vi "rsscope_core_global.vi"() -> ()   [LabVIEW 2018] (continued)
all actions waiting for a trigger event. In particular, *TRG generates a manual trigger signal (Manual Trigger).\n\nAvailable Repeated Capabilities:\nNone\n\nRemote-control command(s):\n*TRG"}, {"Level"=2, "Class Only"=FALSE, "Identifier"="RSSCOPE_ATTR_SEND_SW_TRIGGER_AND_WAIT", "Descriptive Name"="Send SW Trigger And Wait", "Data Type"=4, "Command"="*TRG", "Access"=1, "Range Table"="", "Read Callback"="", "Write Callback"="", "Supported Models"="", "Instrument Options"="", "Flags"=1, "Help"="Triggers all actions waiting for a trigger event. In particular, *TRG generates a manual trigger signal (Manual Trigger). This attribute waits for operation complete.\n\nAvailable Repeated Capabilities:\nNone\n\nRemote-control command(s):\n*TRG"}, {"Level"=1, "Class Only"=TRUE, "Identifier"="", "Descriptive Name"="Cursors", "Data Type"=0, "Command"="", "Access"=0, "Range Table"="", "Read Callback"="", "Write Callback"="", "Supported Models"="", "Instrument Options"="", "Flags"=0, "Help"="Cursor measurements determine the results at the current cursor positions. The cursors can be positioned manually or can be configured to follow the peaks of the waveform. Up to four sets of cursors can be configured and displayed. Each set of cursors consists of a pair of horizontal or vertical cursors, or both. Cursors can be coupled so that the initially defined distance is always maintained."}, {"Level"=2, "Class Only"=FALSE, "Identifier"="RSSCOPE_ATTR_CURSOR_ENABLED", "Descriptive Name"="Cursor Enabled", "Data Type"=3, "Command"="CURS{Cursor}:STAT", "Access"=2, "Range Table"="", "Read Callback"="", "Write Callback"="", "Supported Models"="", "Instrument Options"="", "Flags"=0, "Help"="Switches the indicated cursor on or off.\n\nAvailable Repeated Capabilities:\nCursor: C1, C2, C3, C4\r\n\nRemote-control command(s):\nCURSor<m>:STATe"}, {"Level"=2, "Class Only"=FALSE, "Identifier"="RSSCOPE_ATTR_ALL_CURSORS_OFF", "Descriptive Name"="All Cursors Off", "Data Type"=4, "Command"="CURS1:AOFF", "Access"=1, "Range Table"="", "Read Callback"="", "Write Callback"="", "Supported Models"="", "Instrument Options"="", "Flags"=0, "Help"="Switches all cursors off.\n\nAvailable Repeated Capabilities:\nNone\n\nRemote-control command(s):\nCURSor<m>:AOFF"}, {"Level"=2, "Class Only"=FALSE, "Identifier"="RSSCOPE_ATTR_CURSOR_MEASUREMENT_TYPE", "Descriptive Name"="Cursor Measurement Type", "Data Type"=0, "Command"="CURS{Cursor}:FUNC", "Access"=2, "Range Table"="rsscope_rngCursorFunction", "Read Callback"="", "Write Callback"="", "Supported Models"="", "Instrument Options"="", "Flags"=0, "Help"="Defines the cursor measurement type.\n\nAvailable Repeated Capabilities:\nCursor: C1, C2, C3, C4\r\n\nRemote-control command(s):\nCURSor<m>:FUNCtion"}, {"Level"=2, "Class Only"=FALSE, "Identifier"="RSSCOPE_ATTR_CURSOR_SOURCE", "Descriptive Name"="Cursor Source", "Data Type"=0, "Command"="CURS{Cursor}:SOUR", "Access"=2, "Range Table"="RsScope_rngCursorSource", "Read Callback"="", "Write Callback"="", "Supported Models"="", "Instrument Options"="", "Flags"=0, "Help"="Defines the source of the cursor measurement.\n\nAvailable Repeated Capabilities:\nCursor: C1, C2, C3, C4\r\n\nRemote-control command(s):\nCURSor<m>:SOURce"}, {"Level"=2, "Class Only"=FALSE, "Identifier"="RSSCOPE_ATTR_CURSOR_TRACKING", "Descriptive Name"="Cursor Tracking", "Data Type"=3, "Command"="CURS{Cursor}:TRAC", "Access"=2, "Range Table"="", "Read Callback"="", "Write Callback"="", "Supported Models"="", "Instrument Options"="", "Flags"=0, "Help"="If set to ON, the horizontal cursor lines follow the waveform.\n\nAvailable Repeated Capabilities:\nCursor: C1, C2, C3, C4\r\n\nRemote-control command(s):\nCURSor<m>:TRACking[:STATe]"}, {"Level"=2, "Class Only"=FALSE, "Identifier"="RSSCOPE_ATTR_CURSOR_RESULT_TABLE_POSITION", "Descriptive Name"="Cursor Result Table Position", "Data Type"=0, "Command"="DISP:RES:CUP", "Access"=2, "Range Table"="RsScope_rngDisplayResultTableDefaultPosition", "Read Callback"="", "Write Callback"="", "Supported Models"="", "Instrument Options"="", "Flags"=0, "Help"="Defines the position of the cursor measurement results on the screen.\n\nAvailable Repeated Capabilities:\nNone\n\nRemote-control command(s):\nDISPlay:RESultboxes:CUPosition"}, {"Level"=2, "Class Only"=FALSE, "Identifier"="RSSCOPE_ATTR_CURSOR_X_POSITION_COUPLING", "Descriptive Name"="Cursor X Position Coupling", "Data Type"=3, "Command"="CURS{Cursor}:XCO", "Access"=2, "Range Table"="", "Read Callback"="", "Write Callback"="", "Supported Models"="", "Instrument Options"="", "Flags"=0, "Help"="Defines the positioning mode of the vertical cursor. \nON: Moving one cursor line moves the other cursor line too. The cursor lines always remain a fixed distance.\nOFF: Each cursor line is positioned independently.\n\nAvailable Repeated Capabilities:\nCursor: C1, C2, C3, C4\r\n\nRemote-control command(s):\nCURSor<m>:XCOupling"}, {"Level"=2, "Class Only"=FALSE, "Identifier"="RSSCOPE_ATTR_CURSOR_Y_POSITION_COUPLING", "Descriptive Name"="Cursor Y Position Coupling", "Data Type"=3, "Command"="CURS{Cursor}:YCO", "Access"=2, "Range Table"="", "Read Callback"="", "Write Callback"="", "Supported Models"="", "Instrument Options"="", "Flags"=0, "Help"="Defines the positioning mode of the horizontal cursor. If the horizontal cursor lines track the waveform, the y-coupling is irrelevant.\nON: Moving one cursor line moves the other cursor line too. The cursor lines always remain a fixed distance.\nOFF: Each cursor line is positioned independently.\n\nAvailable Repeated Capabilities:\nCursor: C1, C2, C3, C4\r\n\nRemote-control command(s):\nCURSor<m>:YCOupling"}, {"Level"=2, "Class Only"=FALSE, "Identifier"="RSSCOPE_ATTR_CURSOR_ENVELOPE_CURVE_1", "Descriptive Name"="Cursor Envelope Curve 1", "Data Type"=0, "Command"="CURS{Cursor}:X1EN", "Access"=2, "Range Table"="rsscope_rngMinMax", "Read Callback"="", "Write Callback"="", "Supported Models"="", "Instrument Options"="", "Flags"=0, "Help"="If the waveform arithmetics are set to envelope curve and cursor tracking is set to &apos;ON&apos;, this setting defines how the first horizontal cursor is positioned.\n\nAvailable Repeated Capabilities:\nCursor: C1, C2, C3, C4\r\n\nRemote-control command(s):\nCURSor<m>:X1ENvelope"}, {"Level"=2, "Class Only"=FALSE, "Identifier"="RSSCOPE_ATTR_CURSOR_ENVELOPE_CURVE_2", "Descriptive Name"="Cursor Envelope Curve 2", "Data Type"=0, "Command"="CURS{Cursor}:X2EN", "Access"=2, "Range Table"="rsscope_rngMinMax", "Read Callback"="", "Write Callback"="", "Supported Models"="", "Instrument Options"="", "Flags"=0, "Help"="If the waveform arithmetics are set to envelope curve and cursor tracking is set to &apos;ON&apos;, this setting defines how the second horizontal cursor is positioned.\n\nAvailable Repeated Capabilities:\nCursor: C1, C2, C3, C4\r\n\nRemote-control command(s):\nCURSor<m>:X2ENvelope"}, {"Level"=2, "Class Only"=FALSE, "Identifier"="RSSCOPE_ATTR_CURSOR_HORIZONTAL_DISTANCE", "Descriptive Name"="Cursor Horizontal Distance", "Data Type"=1, "Command"="CURS{Cursor}:YDEL?", "Access"=0, "Range Table"="", "Read Callback"="", "Write Callback"="", "Supported Models"="", "Instrument Options"="", "Flags"=0, "Help"="Queries the delta value (distance) of the two horizontal cursor lines.\n\nAvailable Repeated Capabilities:\nCursor: C1, C2, C3, C4\r\n\nRemote-control command(s):\nCURSor<m>:YDELta[:VALue]?"}, {"Level"=2, "Class Only"=FALSE, "Identifier"="RSSCOPE_ATTR_CURSOR_HORIZONTAL_DELTA_SLOPE", "Descriptive Name"="Cursor Horizontal Delta Slope", "Data Type"=1, "Command"="CURS{Cursor}:YDEL:SLOP?", "Access"=0, "Range Table"="", "Read Callback"="", "Write Callback"="", "Supported Models"="", "Instrument Options"="", "Flags"=0, "Help"="Returns the inverse value of the voltage difference - the reciprocal of the vertical distance of two horizontal cursor lines: 1/delta_V.\n\nAvailable Repeated Capabilities:\nCursor: C1, C2, C3, C4\r\n\nRemote-control command(s):\nCURSor<m>:YDELta:SLOPe?"}, {"Level"=2, "Class Only"=FALSE, "Identifier"="RSSCOPE_ATTR_CURSOR_VERTICAL_DISTANCE", "Descriptive Name"="Cursor Vertical Distance", "Data Type"=1, "Command"="CURS{Cursor}:XDEL?", "Access"=0, "Range Table"="", "Read Callback"="", "Write Callback"="", "Supported Models"="", "Instrument Options"="", "Flags"=0, "Help"="Queries the delta value (distance) of two vertical cursor lines.\n\nAvailable Repeated Capabilities:\nCursor: C1, C2, C3, C4\r\n\nRemote-control command(s):\nCURSor<m>:XDELta[:VALue]?"}, {"Level"=2, "Class Only"=FALSE, "Identifier"="RSSCOPE_ATTR_CURSOR_INVERSE_DISTANCE", "Descriptive Name"="Cursor Inverse Distance", "Data Type"=1, "Command"="CURS{Cursor}:XDEL:INV?", "Access"=0, "Range Table"="", "Read Callback"="", "Write Callback"="", "Supported Models"="", "Instrument Options"="", "Flags"=0, "Help"="Queries the inverse value of the delta value (distance) of the two vertical cursor lines.\n\nAvailable Repeated Capabilities:\nCursor: C1, C2, C3, C4\r\n\nRemote-control command(s):\nCURSor<m>:XDELta:INVerse?"}, {"Level"=2, "Class Only"=FALSE, "Identifier"="RSSCOPE_ATTR_CURSOR_SEARCH_PEAK", "Descriptive Name"="Cursor Search Peak", "Data Type"=4, "Command"="CURS{Cursor}:MAX", "Access"=1, "Range Table"="", "Read Callback"="", "Write Callback"="", "Supported Models"="", "Instrument Options"="", "Flags"=0, "Help"="Sets both cursors to the absolute peak value.\n\nAvailable Repeated Capabilities:\nCursor: C1, C2, C3, C4\r\n\nRemote-control command(s):\nCURSor<m>:MAXimum[:PEAK]"}, {"Level"=2, "Class Only"=FALSE, "Identifier"="RSSCOPE_ATTR_CURSOR_SEARCH_NEXT_LEFT", "Descriptive Name"="Cursor Search Next Left", "Data Type"=4, "Command"="CURS{Cursor}:MAX:LEFT", "Access"=1, "Range Table"="", "Read Callback"="", "Write Callback"="", "Supported Models"="", "Instrument Options"="", "Flags"=0, "Help"="Sets cursor 2 to the next maximum to the left of the current position.\n\nAvailable Repeated Capabilities:\nCursor: C1, C2, C3, C4\r\n\nRemote-control command(s):\nCURSor<m>:MAXimum:LEFT"}, {"Level"=2, "Class Only"=FALSE, "Identifier"="RSSCOPE_ATTR_CURSOR_SEARCH_NEXT_RIGHT", "Descriptive Name"="Cursor Search Next Right", "Data Type"=4, "Command"="CURS{Cursor}:MAX:RIGH", "Access"=1, "Range Table"="", "Read Callback"="", "Write Callback"="", "Supported Models"="", "Instrument Options"="", "Flags"=0, "Help"="Sets cursor 2 to the next peak to the right (from the current position).\n\nAvailable Repeated Capabilities:\nCursor: C1, C2, C3, C4\r\n\nRemote-control command(s):\nCURSor<m>:MAXimum:RIGHt"}, {"Level"=2, "Class Only"=FALSE, "Identifier"="RSSCOPE_ATTR_CURSOR_SEARCH_NEXT_ABSOLUTE", "Descriptive Name"="Cursor Search Next Absolute", "Data Type"=4, "Command"="CURS{Cursor}:MAX:NEXT", "Access"=1, "Range Table"="", "Read Callback"="", "Write Callback"="", "Supported Models"="", "Instrument Options"="", "Flags"=0, "Help"="Sets cursor 2 to the next smaller peak (from the current position).\n\nAvailable Repeated Capabilities:\nCursor: C1, C2, C3, C4\r\n\nRemote-control command(s):\nCURSor<m>:MAXimum:NEXT"}, {"Level"=2, "Class Only"=FALSE, "Identifier"="RSSCOPE_ATTR_CURSOR_PEAK_EXCURSION", "Descriptive Name"="Cursor Peak Excursion", "Data Type"=0, "Command"="CURS{Cursor}:PEXC", "Access"=2, "Range Table"="rsscope_rngPeakExcursion", "Read Callback"="", "Write Callback"="", "Supported Models"="", "Instrument Options"="", "Flags"=0, "Help"="Defines the minimum level by which the waveform must rise or fall so that it will be identified as a maximum or a minimum by the search functions.\n\nAvailable Repeated Capabilities:\nCursor: C1, C2, C3, C4\r\n\nRemote-control command(s):\nCURSor<m>:PEXCursion"}, {"Level"=2, "Class Only"=FALSE, "Identifier"="RSSCOPE_ATTR_CURSOR_THRESHOLD", "Descriptive Name"="Cursor Threshold", "Data Type"=1, "Command"="CURS{Cursor}:THR", "Access"=2, "Range Table"="", "Read Callback"="", "Write Callback"="", "Supported Models"="", "Instrument Options"="", "Flags"=0, "Help"="Defines an absolute threshold as an additional condition for the peak search. Only peaks that exceed the threshold are detected.\n\nAvailable Repeated Capabilities:\nCursor: C1, C2, C3, C4\r\n\nRemote-control command(s):\nCURSor<m>:THReshold"}, {"Level"=2, "Class Only"=FALSE, "Identifier"="RSSCOPE_ATTR_CURSOR_SOURCE_2", "Descriptive Name"="Cursor Source 2", "Data Type"=0, "Command"="CURS{Cursor}:SSO", "Access"=2, "Range Table"="RsScope_rngCursorSource", "Read Callback"="", "Write Callback"="", "Supported Models"="", "Instrument Options"="", "Flags"=0, "Help"="Selects the second cursor source.\n\nAvailable Repeated Capabilities:\nCursor: C1, C2, C3, C4\r\n\nRemote-control command(s):\nCURSor<m>:SSOurce"}, {"Level"=2, "Class Only"=FALSE, "Identifier"="RSSCOPE_ATTR_CURSOR_SOURCE_2_ENABLED", "Descriptive Name"="Cursor Source 2 Enabled", "Data Type"=3, "Command"="CURS{Cursor}:USS", "Access"=2, "Range Table"="", "Read Callback"="", "Write Callback"="", "Supported Models"="", "Instrument Options"="", "Flags"=0, "Help"="Enables the second cursor source.\nIf enabled, the second corsor lines Cx.2 measure on the second source. Using a second source, you can measure differences between two channels with cursors.\n\nAvailable Repeated Capabilities:\nCursor: C1, C2, C3, C4\r\n\nRemote-control command(s):\nCURSor<m>:USSource"}, {"Level"=2, "Class Only"=FALSE, "Identifier"="RSSCOPE_ATTR_CURSOR_LABEL_ENABLED", "Descriptive Name"="Cursor Label Enabled", "Data Type"=3, "Command"="CURS{Cursor}:LAB", "Access"=2, "Range Table"="", "Read Callback"="", "Write Callback"="", "Supported Models"="", "Instrument Options"="", "Flags"=0, "Help"="Shows the cursor labels in the diagram.\n\nAvailable Repeated Capabilities:\nCursor: C1, C2, C3, C4\r\n\nRemote-control command(s):\nCURSor<m>:LABel"}, {"Level"=2, "Class Only"=FALSE, "Identifier"="RSSCOPE_ATTR_CURSOR_STYLE", "Descriptive Name"="Cursor Style", "Data Type"=0, "Command"="CURS{Cursor}:STYL", "Access"=2, "Range Table"="RsScope_rngCursorStyle", "Read Callback"="", "Write Callback"="", "Supported Models"="", "Instrument Options"="", "Flags"=0, "Help"="Defines how the cursor is displayed in the diagram.\n\nAvailable Repeated Capabilities:\nCursor: C1, C2, C3, C4\r\n\nRemote-control command(s):\nCURSor<m>:STYLe"}, {"Level"=2, "Class Only"=FALSE, "Identifier"="RSSCOPE_ATTR_CURSOR_SHOW_IN_ALL_DIAGRAMS", "Descriptive Name"="Cursor Show In All Diagrams", "Data Type"=3, "Command"="CURS:SIAD", "Access"=2, "Range Table"="", "Read Callback"="", "Write Callback"="", "Supported Models"="", "Instrument Options"="", "Flags"=0, "Help"="Shows the enabled cursor measurements in all active diagrams of the same domain (time/ spectrum). All cursor measurements are affected.\n\nAvailable Repeated Capabilities:\nNone\n\nRemote-control command(s):\nCURSor<m>:SIAD"}, {"Level"=2, "Class Only"=TRUE, "Identifier"="", "Descriptive Name"="Spectrum Waveforms", "Data Type"=0, "Command"="", "Access"=0, "Range Table"="", "Read Callback"="", "Write Callback"="", "Supported Models"="", "Instrument Options"="", "Flags"=0, "Help"="If the measurement source is a spectrum waveform, the result box provides buttons for easy center definition and peak search."}, {"Level"=3, "Class Only"=FALSE, "Identifier"="RSSCOPE_ATTR_CURSOR_SPECTRUM_WAVEFORMS_C1_TO_CENTER", "Descriptive Name"="Cursor Spectrum Waveforms C1 To Center", "Data Type"=4, "Command"="CURS{Cursor}:FFT:TOC", "Access"=1, "Range Table"="", "Read Callback"="", "Write Callback"="", "Supported Models"="", "Instrument Options"="", "Flags"=0, "Help"="Sets the vertical cursor line c1 to the center frequency.\n\nAvailable Repeated Capabilities:\nCursor: C1, C2, C3, C4\r\n\nRemote-control command(s):\nCURSor<m>:FFT:TOCenter"}, {"Level"=3, "Class Only"=FALSE, "Identifier"="RSSCOPE_ATTR_CURSOR_SPECTRUM_WAVEFORMS_CENTER_TO_C1", "Descriptive Name"="Cursor Spectrum Waveforms Center To C1", "Data Type"=4, "Command"="CURS{Cursor}:FFT:SETC", "Access"=1, "Range Table"="", "Read Callback"="", "Write Callback"="", "Supported Models"="", "Instrument Options"="", "Flags"=0, "Help"="Sets the center frequency to the frequency value that is measured at cursor line c1.\n\nAvailable Repeated Capabilities:\nCursor: C1, C2, C3, C4\r\n\nRemote-control command(s):\nCURSor<m>:FFT:SETCenter"}, {"Level"=2, "Class Only"=TRUE, "Identifier"="", "Descriptive Name"="Cursor Position", "Data Type"=0, "Command"="", "Access"=0, "Range Table"="", "Read Callback"="", "Write Callback"="", "Supported Models"="", "Instrument Options"="", "Flags"=0, "Help"="Selects Cursor Position"}, {"Level"=3, "Class Only"=FALSE, "Identifier"="RSSCOPE_ATTR_CURSOR_X_POSITION", "Descriptive Name"="Cursor X Position", "Data Type"=1, "Command"="CURS{Cursor}:X{CPosition}P", "Access"=2, "Range Table"="", "Read Callback"="", "Write Callback"="", "Supported Models"="", "Instrument Options"="", "Flags"=1, "Help"="Defines the vertical position of selected cursor or cursor line.\n\nValid values for CPosition repeated capability are:\n1 - Lower\n2 - Upper\n\nAvailable Repeated Capabilities:\nCursor: C1, C2, C3, C4\r\nCPosition: P1, P2\r\n\nRemote-control command(s):\nCURSor<m>:X<CPosition>Position"}, {"Level"=3, "Class Only"=FALSE, "Identifier"="RSSCOPE_ATTR_CURSOR_Y_POSITION", "Descriptive Name"="Cursor Y Position", "Data Type"=1, "Command"="CURS{Cursor}:Y{CPosition}P", "Access"=2, "Range Table"="", "Read Callback"="", "Write Callback"="", "Supported Models"="", "Instrument Options"="", "Flags"=1, "Help"="Defines the horizontal position of selected cursor or cursor line.\n\nValid values for CPosition repeated capability are:\n1 - Lower\n2 - Upper\n\nAvailable Repeated Capabilities:\nCursor: C1, C2, C3, C4\r\nCPosition: P1, P2\r\n\nRemote-control command(s):\nCURSor<m>:Y<CPosition>Position"}, {"Level"=1, "Class Only"=TRUE, "Identifier"="", "Descriptive Name"="Measurements", "Data Type"=0, "Command"="", "Access"=0, "Range Table"="", "Read Callback"="", "Write Callback"="", "Supported Models"="", "Instrument Options"="", "Flags"=0, "Help"="Configures scope measurements and queries results."}, {"Level"=2, "Class Only"=TRUE, "Identifier"="", "Descriptive Name"="General Measurement Settings", "Data Type"=0, "Command"="", "Access"=0, "Range Table"="", "Read Callback"="", "Write Callback"="", "Supported Models"="", "Instrument Options"="", "Flags"=0, "Help"="Settings common for all measurements."}, {"Level"=3, "Class Only"=FALSE, "Identifier"="RSSCOPE_ATTR_MEASUREMENT_ENABLED", "Descriptive Name"="Measurement Enabled", "Data Type"=3, "Command"="MEAS{Measurement}", "Access"=2, "Range Table"="", "Read Callback"="", "Write Callback"="", "Supported Models"="", "Instrument Options"="", "Flags"=1, "Help"="Switches the indicated measurement on or off.\n\nAvailable Repeated Capabilities:\nMeasurement: Meas1, Meas2, Meas3, Meas4, Meas5, Meas6, Meas7, Meas8, Meas9, Meas10\r\n\nRemote-control command(s):\nMEASurement<m>[:ENABle]"}, {"Level"=3, "Class Only"=FALSE, "Identifier"="RSSCOPE_ATTR_MULTIPLE_MEASUREMENT_ENABLED", "Descriptive Name"="Multiple Measurement Enabled", "Data Type"=3, "Command"="MEAS{Measurement}:MULT", "Access"=2, "Range Table"="", "Read Callback"="", "Write Callback"="", "Supported Models"="", "Instrument Options"="", "Flags"=0, "Help"="The measurement is performed repeatedly if the measured parameter occurs several times inside the defined gate.\n\nAvailable Repeated Capabilities:\nMeasurement: Meas1, Meas2, Meas3, Meas4, Meas5, Meas6, Meas7, Meas8, Meas9, Meas10\r\n\nRemote-control command(s):\nMEASurement<m>:MULTiple"}, {"Level"=3, "Class Only"=FALSE, "Identifier"="RSSCOPE_ATTR_MULTIPLE_MEASUREMENT_COUNT", "Descriptive Name"="Multiple Measurement Count", "Data Type"=0, "Command"="MEAS{Measurement}:MNOM", "Access"=2, "Range Table"="rsscope_rngMultipleMeasurementCount", "Read Callback"="", "Write Callback"="", "Supported Models"="", "Instrument Options"="", "Flags"=0, "Help"="This function sets the maximum number of measurements per acquisition if multiple measurement is enabled.\n\nAvailable Repeated Capabilities:\nMeasurement: Meas1, Meas2, Meas3, Meas4, Meas5, Meas6, Meas7, Meas8, Meas9, Meas10\r\n\nRemote-control command(s):\nMEASurement<m>:MNOMeas"}, {"Level"=3, "Class Only"=FALSE, "Identifier"="RSSCOPE_ATTR_MEASUREMENT_CATEGORY", "Descriptive Name"="Measurement Category", "Data Type"=0, "Command"="MEAS{Measurement}:CAT", "Access"=2, "Range Table"="rsscope_rngMeasurementCategory", "Read Callback"="", "Write Callback"="", "Supported Models"="", "Instrument Options"="", "Flags"=0, "Help"="Defines the measurement category.\n\nAvailable Repeated Capabilities:\nMeasurement: Meas1, Meas2, Meas3, Meas4, Meas5, Meas6, Meas7, Meas8, Meas9, Meas10\r\n\nRemote-control command(s):\nMEASurement<m>:CATegory"}, {"Level"=3, "Class Only"=FALSE, "Identifier"="RSSCOPE_ATTR_ADDITIONAL_MEASUREMENTS_ENABLE", "Descriptive Name"="Additional Measurements Enable", "Data Type"=4, "Command"="MEAS{Measurement}:AON", "Access"=1, "Range Table"="", "Read Callback"="", "Write Callback"="", "Supported Models"="", "Instrument Options"="", "Flags"=0, "Help"="Enables all additional measurements in all categories of the indicated measurement.\n\nAvailable Repeated Capabilities:\nMeasurement: Meas1, Meas2, Meas3, Meas4, Meas5, Meas6, Meas7, Meas8, Meas9, Meas10\r\n\nRemote-control command(s):\nMEASurement<m>:AON"}, {"Level"=3, "Class Only"=FALSE, "Identifier"="RSSCOPE_ATTR_ADDITIONAL_MEASUREMENTS_DISABLE", "Descriptive Name"="Additional Measurements Disable", "Data Type"=4, "Command"="MEAS{Measurement}:AOFF", "Access"=1, "Range Table"="", "Read Callback"="", "Write Callback"="", "Supported Models"="", "Instrument Options"="", "Flags"=0, "Help"="Disables all additional measurements in all categories of the indicated measurement.\n\nAvailable Repeated Capabilities:\nMeasurement: Meas1, Meas2, Meas3, Meas4, Meas5, Meas6, Meas7, Meas8, Meas9, Meas10\r\n\nRemote-control command(s):\nMEASurement<m>:AOFF"}, {"Level"=3, "Class Only"=FALSE, "Identifier"="RSSCOPE_ATTR_CLEAR_MEASUREMENT_STATISTIC_DATA", "Descriptive Name"="Clear Measurement Statistic Data", "Data Type"=4, "Command"="MEAS{Measurement}:CLE", "Access"=1, "Range Table"="", "Read Callback"="", "Write Callback"="", "Supported Models"="", "Instrument Options"="", "Flags"=0, "Help"="Deletes the statistic results of the indicated mesurement.\n\nAvailable Repeated Capabilities:\nMeasurement: Meas1, Meas2, Meas3, Meas4, Meas5, Meas6, Meas7, Meas8, Meas9, Meas10\r\n\nRemote-control command(s):\nMEASurement<m>:CLEar"}, {"Level"=3, "Class Only"=FALSE, "Identifier"="RSSCOPE_ATTR_MEASUREMENT_LIMIT_TYPE", "Descriptive Name"="Measurement Limit Type", "Data Type"=0, "Command"="MEAS{Measurement}:LCH", "Access"=2, "Range Table"="rsscope_rngLimitType", "Read Callback"="", "Write Callback"="", "Supported Models"="", "Instrument Options"="", "Flags"=0, "Help"="Defines the type of the limit check that can run together with the measurement.\n\nAvailable Repeated Capabilities:\nMeasurement: Meas1, Meas2, Meas3, Meas4, Meas5, Meas6, Meas7, Meas8, Meas9, Meas10\r\n\nRemote-control command(s):\nMEASurement<m>:LCHeck"}, {"Level"=3, "Class Only"=FALSE, "Identifier"="RSSCOPE_ATTR_MEASUREMENT_DISPLAY_STYLE", "Descriptive Name"="Measurement Display Style", "Data Type"=0, "Command"="MEAS{Measurement}:DISP:STYL", "Access"=2, "Range Table"="rsscope_rngDisplayStyle", "Read Callback"="", "Write Callback"="", "Supported Models"="", "Instrument Options"="", "Flags"=0, "Help"="Selects the style in which the measurement waveform is displayed.\n\nAvailable Repeated Capabilities:\nMeasurement: Meas1, Meas2, Meas3, Meas4, Meas5, Meas6, Meas7, Meas8, Meas9, Meas10\r\n\nRemote-control command(s):\nMEASurement<m>:DISPlay:STYLe"}, {"Level"=3, "Class Only"=FALSE, "Identifier"="RSSCOPE_ATTR_GENERATE_BEEP_ON_MEASUREMENT_EVENT", "Descriptive Name"="Generate Beep On Measurement Event", "Data Type"=0, "Command"="MEAS{Measurement}:ONV:BEEP", "Access"=2, "Range Table"="rsscope_rngMeasurementEvent", "Read Callback"="", "Write Callback"="", "Supported Models"="", "Instrument Options"="", "Flags"=0, "Help"="Generates a beep sound for the specified event.\n\nAvailable Repeated Capabilities:\nMeasurement: Meas1, Meas2, Meas3, Meas4, Meas5, Meas6, Meas7, Meas8, Meas9, Meas10\r\n\nRemote-control command(s):\nMEASurement<m>:ONViolation:BEEP"}, {"Level"=3, "Class Only"=FALSE, "Identifier"="RSSCOPE_ATTR_STOP_ACQUISITION_ON_MEASUREMENT_EVENT", "Descriptive Name"="Stop Acquisition On Measurement Event", "Data Type"=0, "Command"="MEAS{Measurement}:ONV:ACQS", "Access"=2, "Range Table"="rsscope_rngMeasurementEvent", "Read Callback"="", "Write Callback"="", "Supported Models"="", "Instrument Options"="", "Flags"=0, "Help"="Stops data acquisition for the specified event.\n\nAvailable Repeated Capabilities:\nMeasurement: Meas1, Meas2, Meas3, Meas4, Meas5, Meas6, Meas7, Meas8, Meas9, Meas10\r\n\nRemote-control command(s):\nMEASurement<m>:ONViolation:ACQStop"}, {"Level"=3, "Class Only"=FALSE, "Identifier"="RSSCOPE_ATTR_PRINT_ON_MEASUREMENT_EVENT", "Descriptive Name"="Print On Measurement Event", "Data Type"=0, "Command"="MEAS{Measurement}:ONV:PRIN", "Access"=2, "Range Table"="rsscope_rngMeasurementEvent", "Read Callback"="", "Write Callback"="", "Supported Models"="", "Instrument Options"="", "Flags"=0, "Help"="Prints a screenshot including the measurement results to the printer defined using SYSTem: COMMunicate: PRINter: SELect<1..2> for the specified event.\n\nAvailable Repeated Capabilities:\nMeasurement: Meas1, Meas2, Meas3, Meas4, Meas5, Meas6, Meas7, Meas8, Meas9, Meas10\r\n\nRemote-control command(s):\nMEASurement<m>:ONViolation:PRINt"}, {"Level"=3, "Class Only"=FALSE, "Identifier"="RSSCOPE_ATTR_SAVE_WAVEFORM_DATA_ON_MEASUREMENT_EVENT", "Descriptive Name"="Save Waveform Data On Measurement Event", "Data Type"=0, "Command"="MEAS{Measurement}:ONV:WFMS", "Access"=2, "Range Table"="rsscope_rngMeasurementEvent", "Read Callback"="", "Write Callback"="", "Supported Models"="", "Instrument Options"="", "Flags"=0, "Help"="Saves the waveform data.\n\nAvailable Repeated Capabilities:\nMeasurement: Meas1, Meas2, Meas3, Meas4, Meas5, Meas6, Meas7, Meas8, Meas9, Meas10\r\n\nRemote-control command(s):\nMEASurement<m>:ONViolation:WFMSave"}, {"Level"=3, "Class Only"=FALSE, "Identifier"="RSSCOPE_ATTR_CREATE_TRIGGER_OUT_PULSE", "Descriptive Name"="Create Trigger Out Pulse", "Data Type"=0, "Command"="MEAS{Measurement}:ONV:TRIG", "Access"=2, "Range Table"="rsscope_rngMeasurementEvent", "Read Callback"="", "Write Callback"="", "Supported Models"="", "Instrument Options"="", "Flags"=0, "Help"="Creates a trigger out pulse on limit or margin violation or on successful completion of themeasurement.\n\nAvailable Repeated Capabilities:\nMeasurement: Meas1, Meas2, Meas3, Meas4, Meas5, Meas6, Meas7, Meas8, Meas9, Meas10\r\n\nRemote-control command(s):\nMEASurement<m>:ONViolation:TRIGgerout"}, {"Level"=3, "Class Only"=FALSE, "Identifier"="RSSCOPE_ATTR_SAVE_REPORT_ON_MEASUREMENT_EVENT", "Descriptive Name"="Save Report On Measurement Event", "Data Type"=0, "Command"="MEAS{Measurement}:ONV:REP", "Access"=2, "Range Table"="rsscope_rngMeasurementEvent", "Read Callback"="", "Write Callback"="", "Supported Models"="", "Instrument Options"="", "Flags"=0, "Help"="Creates and saves a report of the current settings and results.\n\nAvailable Repeated Capabilities:\nMeasurement: Meas1, Meas2, Meas3, Meas4, Meas5, Meas6, Meas7, Meas8, Meas9, Meas10\r\n\nRemote-control command(s):\nMEASurement<m>:ONViolation:REPort"}, {"Level"=3, "Class Only"=FALSE, "Identifier"="RSSCOPE_ATTR_START_EXTERNAL_APPLICATION_ON_MEASUREMENT_EVENT", "Descriptive Name"="Start External Application On Measurement Event", "Data Type"=0, "Command"="MEAS{Measurement}:ONV:RUN", "Access"=2, "Range Table"="rsscope_rngMeasurementEvent", "Read Callback"="", "Write Callback"="", "Supported Models"="", "Instrument Options"="", "Flags"=0, "Help"="Starts an external application.\n\nAvailable Repeated Capabilities:\nMeasurement: Meas1, Meas2, Meas3, Meas4, Meas5, Meas6, Meas7, Meas8, Meas9, Meas10\r\n\nRemote-control command(s):\nMEASurement<m>:ONViolation:RUNexec"}, {"Level"=3, "Class Only"=FALSE, "Identifier"="RSSCOPE_ATTR_MEASUREMENT_PREFIX_ENABLED", "Descriptive Name"="Measurement Prefix Enabled", "Data Type"=3, "Command"="MEAS{Measurement}:ARN", "Access"=2, "Range Table"="", "Read Callback"="", "Write Callback"="", "Supported Models"="", "Instrument Options"="", "Flags"=0, "Help"="Enables a prefix that indicates the measurement type in the result string of the MEASurement<m>: ARES? command.\n\nAvailable Repeated Capabilities:\nMeasurement: Meas1, Meas2, Meas3, Meas4, Meas5, Meas6, Meas7, Meas8, Meas9, Meas10\r\n\nRemote-control command(s):\nMEASurement<m>:ARNames"}, {"Level"=3, "Class Only"=FALSE, "Identifier"="RSSCOPE_ATTR_DEFINE_FIRST_MEASUREMENT_SOURCE", "Descriptive Name"="Define First Measurement Source", "Data Type"=0, "Command"="MEAS{Measurement}:FSRC", "Access"=2, "Range Table"="rsscope_rngWaveformParameter", "Read Callback"="", "Write Callback"="", "Supported Models"="", "Instrument Options"="", "Flags"=0, "Help"="Defines the first measurement source. The command is an alternative to MEASurement<m>:SOURce.\n\nAvailable Repeated Capabilities:\nMeasurement: Meas1, Meas2, Meas3, Meas4, Meas5, Meas6, Meas7, Meas8, Meas9, Meas10\r\n\nRemote-control command(s):\nMEASurement<m>:FSRC"}, {"Level"=3, "Class Only"=FALSE, "Identifier"="RSSCOPE_ATTR_DEFINE_SECOND_MEASUREMENT_SOURCE", "Descriptive Name"="Define Second Measurement Source", "Data Type"=0, "Command"="MEAS{Measurement}:SSRC", "Access"=2, "Range Table"="rsscope_rngWaveformParameter", "Read Callback"="", "Write Callback"="", "Supported Models"="", "Instrument Options"="", "Flags"=0, "Help"="Defines the second measurement source. The command is an alternative to MEASurement<m>:SOURce.\n\nAvailable Repeated Capabilities:\nMeasurement: Meas1, Meas2, Meas3, Meas4, Meas5, Meas6, Meas7, Meas8, Meas9, Meas10\r\n\nRemote-control command(s):\nMEASurement<m>:SSRC"}, {"Level"=2, "Class Only"=TRUE, "Identifier"="", "Descriptive Name"="Amplitude vs. Time Measurement", "Data Type"=0, "Command"="", "Access"=0, "Range Table"="", "Read Callback"="", "Write Callback"="", "Supported Models"="", "Instrument Options"="", "Flags"=0, "Help"="Contains Amplitude vs. Time measurement settings."}, {"Level"=3, "Class Only"=FALSE, "Identifier"="RSSCOPE_ATTR_AMPT_MAIN_MEASUREMENT", "Descriptive Name"="Amplitude Time Main Measurement", "Data Type"=0, "Command"="MEAS{Measurement}:MAIN", "Access"=2, "Range Table"="rsscope_rngAmplitudeTimeMeasurementType", "Read Callback"="", "Write Callback"="", "Supported Models"="", "Instrument Options"="", "Flags"=1, "Help"="Defines or queries the main measurement. This measurement is the one referred to if the measurement waveform is used as a source for math calculations. The main measurement type must belong to the same category as the other types assigned to the same measurement waveform, if there are any.\n\nAvailable Repeated Capabilities:\nMeasurement: Meas1, Meas2, Meas3, Meas4, Meas5, Meas6, Meas7, Meas8, Meas9, Meas10\r\n\nRemote-control command(s):\nMEASurement<m>:MAIN"}, {"Level"=3, "Class Only"=FALSE, "Identifier"="RSSCOPE_ATTR_AMPT_AREA_LEVEL", "Descriptive Name"="Amplitude Time Area Level", "Data Type"=1, "Command"="MEAS{Measurement}:AMPT:ALEV", "Access"=2, "Range Table"="", "Read Callback"="", "Write Callback"="", "Supported Models"="", "Instrument Options"="", "Flags"=0, "Help"="Defines the reference level used to integrate the waveform.\n\nAvailable Repeated Capabilities:\nMeasurement: Meas1, Meas2, Meas3, Meas4, Meas5, Meas6, Meas7, Meas8, Meas9, Meas10\r\n\nRemote-control command(s):\nMEASurement<m>:AMPTime:ALEVel"}, {"Level"=3, "Class Only"=FALSE, "Identifier"="RSSCOPE_ATTR_AMPT_SIGNAL_DETECTION_THRESHOLD", "Descriptive Name"="Amplitude Time Signal Detection Threshold", "Data Type"=0, "Command"="MEAS{Measurement}:DETT", "Access"=2, "Range Table"="rsscope_rngSignalDetectionThreshold", "Read Callback"="", "Write Callback"="", "Supported Models"="", "Instrument Options"="", "Flags"=0, "Help"="Defines the value above which measurement results are displayed. Values beneath the threshold are considered to be noise and are ignored.\n\nAvailable Repeated Capabilities:\nMeasurement: Meas1, Meas2, Meas3, Meas4, Meas5, Meas6, Meas7, Meas8, Meas9, Meas10\r\n\nRemote-control command(s):\nMEASurement<m>:DETThreshold"}, {"Level"=3, "Class Only"=FALSE, "Identifier"="RSSCOPE_ATTR_AMPLITUDE_PULSES_SLOPE", "Descriptive Name"="Amplitude Pulses Slope", "Data Type"=0, "Command"="MEAS{Measurement}:AMPT:PSL", "Access"=2, "Range Table"="rsscope_rngTriggerSlope", "Read Callback"="", "Write Callback"="", "Supported Models"="", "Instrument Options"="", "Flags"=0, "Help"="Sets the first slope of the pulses to be counted.\n\nAvailable Repeated Capabilities:\nMeasurement: Meas1, Meas2, Meas3, Meas4, Meas5, Meas6, Meas7, Meas8, Meas9, Meas10\r\n\nRemote-control command(s):\nMEASurement<m>:AMPTime:PSLope"}, {"Level"=3, "Class Only"=FALSE, "Identifier"="RSSCOPE_ATTR_AMPLITUDE_MEASURED_SLOPE", "Descriptive Name"="Amplitude Measured Slope", "Data Type"=0, "Command"="MEAS{Measurement}:AMPT:PFSL", "Access"=2, "Range Table"="rsscope_rngAmplitudeMeasuredSlope", "Read Callback"="", "Write Callback"="", "Supported Models"="", "Instrument Options"="", "Flags"=0, "Help"="Selects the slope direction for frequency and period measurements.\n\nAvailable Repeated Capabilities:\nMeasurement: Meas1, Meas2, Meas3, Meas4, Meas5, Meas6, Meas7, Meas8, Meas9, Meas10\r\n\nRemote-control command(s):\nMEASurement<m>:AMPTime:PFSLope"}, {"Level"=3, "Class Only"=FALSE, "Identifier"="RSSCOPE_ATTR_AMPLITUDE_EDGES_SLOPE", "Descriptive Name"="Amplitude Edges Slope", "Data Type"=0, "Command"="MEAS{Measurement}:AMPT:ESL", "Access"=2, "Range Table"="rsscope_rngTriggerSlope", "Read Callback"="", "Write Callback"="", "Supported Models"="", "Instrument Options"="", "Flags"=0, "Help"="Sets the edge direction to be counted: rising edges, falling edges, or both.\n\nAvailable Repeated Capabilities:\nMeasurement: Meas1, Meas2, Meas3, Meas4, Meas5, Meas6, Meas7, Meas8, Meas9, Meas10\r\n\nRemote-control command(s):\nMEASurement<m>:AMPTime:ESLope"}, {"Level"=3, "Class Only"=FALSE, "Identifier"="RSSCOPE_ATTR_AMPLITUDE_CLOCK_SLOPE", "Descriptive Name"="Amplitude Clock Slope", "Data Type"=0, "Command"="MEAS{Measurement}:AMPT:CSL", "Access"=2, "Range Table"="rsscope_rngTriggerSlope", "Read Callback"="", "Write Callback"="", "Supported Models"="", "Instrument Options"="", "Flags"=0, "Help"="Sets the edge of the clock from which the setup and hold times are measured.\n\nAvailable Repeated Capabilities:\nMeasurement: Meas1, Meas2, Meas3, Meas4, Meas5, Meas6, Meas7, Meas8, Meas9, Meas10\r\n\nRemote-control command(s):\nMEASurement<m>:AMPTime:CSLope"}, {"Level"=3, "Class Only"=FALSE, "Identifier"="RSSCOPE_ATTR_AMPLITUDE_TIME_DATA_REFERENCE_LEVEL", "Descriptive Name"="Amplitude Time Data Reference Level", "Data Type"=0, "Command"="MEAS{Measurement}:AMPT:DATA:LSEL", "Access"=2, "Range Table"="rsscope_rngAmpRefLevSelection", "Read Callback"="", "Write Callback"="", "Supported Models"="", "Instrument Options"="", "Flags"=0, "Help"="Selects the reference level of the data on which the setup and hold time are measured.\n\nAvailable Repeated Capabilities:\nMeasurement: Meas1, Meas2, Meas3, Meas4, Meas5, Meas6, Meas7, Meas8, Meas9, Meas10\r\n\nRemote-control command(s):\nMEASurement<m>:AMPTime:DATA<n>:LSELect"}, {"Level"=3, "Class Only"=FALSE, "Identifier"="RSSCOPE_ATTR_AMPLITUDE_TIME_CLOCK_REFERENCE_LEVEL", "Descriptive Name"="Amplitude Time Clock Reference Level", "Data Type"=0, "Command"="MEAS{Measurement}:AMPT:CLCK:LSEL", "Access"=2, "Range Table"="rsscope_rngAmpRefLevSelection", "Read Callback"="", "Write Callback"="", "Supported Models"="", "Instrument Options"="", "Flags"=0, "Help"="Selects the reference level of the clock on which the time is measured. Reference level and clock slope define the time point for setup and hold measurements.\n\nAvailable Repeated Capabilities:\nMeasurement: Meas1, Meas2, Meas3, Meas4, Meas5, Meas6, Meas7, Meas8, Meas9, Meas10\r\n\nRemote-control command(s):\nMEASurement<m>:AMPTime:CLCK<n>:LSELect"}, {"Level"=3, "Class Only"=FALSE, "Identifier"="RSSCOPE_ATTR_AMPT_PULSE_TRAIN_COUNT", "Descriptive Name"="Amplitude Pulse Train Count", "Data Type"=0, "Command"="MEAS{Measurement}:AMPT:PTC", "Access"=2, "Range Table"="rsscope_rngAmpPulseTrain", "Read Callback"="", "Write Callback"="", "Supported Models"="", "Instrument Options"="", "Flags"=0, "Help"="Sets the number of positive pulses for the pulse train measurement. It measures the duration of N positive pulses from the rising edge of the first pulse to the falling edge of the N-th pulse.\n\nAvailable Repeated Capabilities:\nMeasurement: Meas1, Meas2, Meas3, Meas4, Meas5, Meas6, Meas7, Meas8, Meas9, Meas10\r\n\nRemote-control command(s):\nMEASurement<m>:AMPTime:PTCount"}, {"Level"=3, "Class Only"=FALSE, "Identifier"="RSSCOPE_ATTR_ENVELOPE_SELECTION", "Descriptive Name"="Envelope Selection", "Data Type"=0, "Command"="MEAS{Measurement}:ENVS", "Access"=2, "Range Table"="rsscope_rngEnvelopeType", "Read Callback"="", "Write Callback"="", "Supported Models"="", "Instrument Options"="", "Flags"=0, "Help"="This attribute selects the envelope.\n\nNote(s):\n(1) This setting is only relevant for measurements on envelope waveforms.\n\nAvailable Repeated Capabilities:\nMeasurement: Meas1, Meas2, Meas3, Meas4, Meas5, Meas6, Meas7, Meas8, Meas9, Meas10\r\n\nRemote-control command(s):\nMEASurement<m>:ENVSelect"}, {"Level"=3, "Class Only"=FALSE, "Identifier"="RSSCOPE_ATTR_AMPLITUDE_DELAY_TO_TRIGGER_SLOPE", "Descriptive Name"="Amplitude Delay To Trigger Slope", "Data Type"=0, "Command"="MEAS{Measurement}:AMPT:DTOT:SLOP", "Access"=2, "Range Table"="rsscope_rngTriggerSlope", "Read Callback"="", "Write Callback"="", "Supported Models"="", "Instrument Options"="", "Flags"=0, "Help"="Sets the edge direction to be used for delay measurement.\n\nAvailable Repeated Capabilities:\nMeasurement: Meas1, Meas2, Meas3, Meas4, Meas5, Meas6, Meas7, Meas8, Meas9, Meas10\r\n\nRemote-control command(s):\nMEASurement<m>:AMPTime:DTOTrigger<n>:SLOPe"}, {"Level"=3, "Class Only"=FALSE, "Identifier"="RSSCOPE_ATTR_AMPLITUDE_DELAY_TO_TRIGGER_REFERENCE_LEVEL", "Descriptive Name"="Amplitude Delay To Trigger Reference Level", "Data Type"=0, "Command"="MEAS{Measurement}:AMPT:DTOT:LSEL", "Access"=2, "Range Table"="rsscope_rngAmpRefLevSelection", "Read Callback"="", "Write Callback"="", "Supported Models"="", "Instrument Options"="", "Flags"=0, "Help"="Selects the reference level of the measurement source on which the delay is measured.\n\nAvailable Repeated Capabilities:\nMeasurement: Meas1, Meas2, Meas3, Meas4, Meas5, Meas6, Meas7, Meas8, Meas9, Meas10\r\n\nRemote-control command(s):\nMEASurement<m>:AMPTime:DTOTrigger<n>:LSELect"}, {"Level"=3, "Class Only"=TRUE, "Identifier"="", "Descriptive Name"="Amplitude vs. Time Arithmetic", "Data Type"=0, "Command"="", "Access"=0, "Range Table"="", "Read Callback"="", "Write Callback"="", "Supported Models"="", "Instrument Options"="", "Flags"=0, "Help"="Contains attributes to configure the arithmetic for amplitude/time measurements"}, {"Level"=4, "Class Only"=FALSE, "Identifier"="RSSCOPE_ATTR_AMPLITUDE_TIME_ARITHMETIC_PARAMETER_MEASUREMENT_TYPE", "Descriptive Name"="Amplitude Time Arithmetic Parameter Measurement Type", "Data Type"=0, "Command"="MEAS{Measurement}:AMPT:ARIT:PAR{ArithmeticParameter}:TYPE", "Access"=2, "Range Table"="RsScope_rngArithmeticMeasurementType", "Read Callback"="", "Write Callback"="", "Supported Models"="", "Instrument Options"="", "Flags"=0, "Help"="Sets the type of amplitude arithmetic measurement.\n\nAvailable Repeated Capabilities:\nMeasurement: Meas1, Meas2, Meas3, Meas4, Meas5, Meas6, Meas7, Meas8, Meas9, Meas10\r\nArithmeticParameter: ArithmeticParm1, ArithmeticParm2\r\n\nRemote-control command(s):\nMEASurement<m>:AMPTime:ARIThmetic:PARameter<n>:TYPE"}, {"Level"=4, "Class Only"=FALSE, "Identifier"="RSSCOPE_ATTR_AMPLITUDE_TIME_ARITHMETIC_PARAMETER_AMPTIME_TYPE", 
